vi "Create Occupancy Grid Map.vi"(8 "error in (no error)":errorcluster, 11 "occupancy grid":dbl[][](array[numeric])) -> (0 "error out":errorcluster, 3 "map reference out":refnum<data-value>)   [LabVIEW 2017, in "NI_Robotics_OccupancyGridWorldMap.lvclass"]
doc: "Generates a map in the form of a grid of variables, or cells, that describe the robot environment."
uses:
  <vilib>/robotics/Navigation/shared/WorldMap/OccupancyGridWorldMap/NI_Robotics_OccupancyGridWorldMap.lvclass
  <vilib>/robotics/Navigation/shared/MapNode/OccupancyGridNode/NI_Robotics_OccupancyGridMapNode.lvclass
  <vilib>/robotics/Navigation/shared/WorldMap/OccupancyGridWorldMap/NI_Robotics_OccupancyGridWorldMap.lvclass/NI_Robotics_OccupancyGridWorldMap.ctl
  <vilib>/robotics/Utilities/NI_Robotics Utilities.lvlib
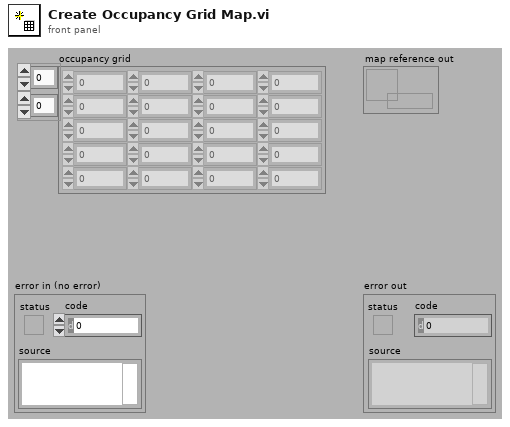
[diagram p1: front panel]
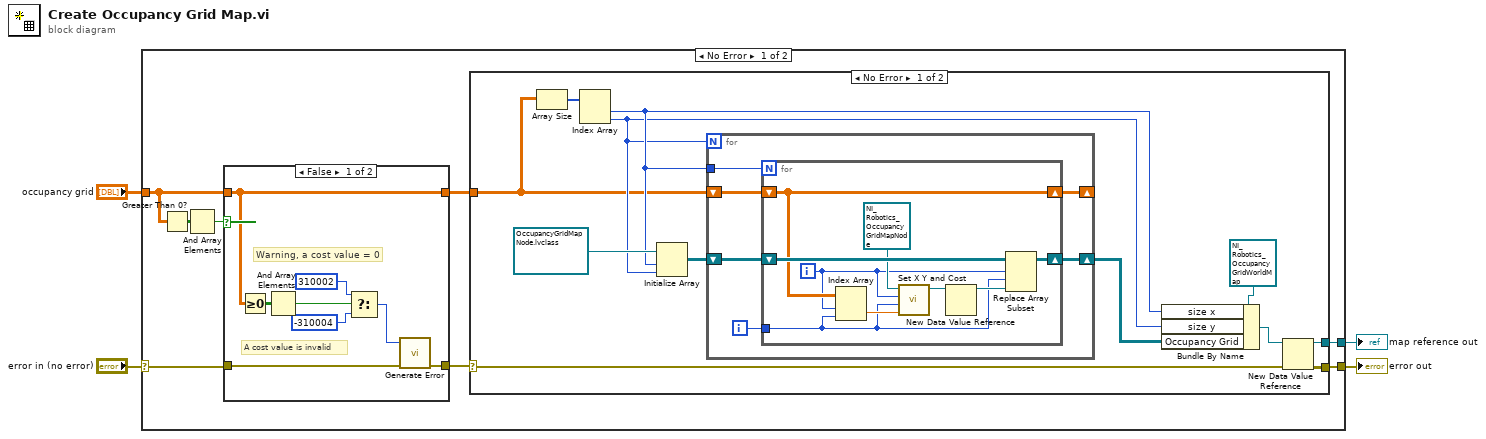
[diagram p0: block diagram]
diagram:
  n1 = case shown="No Error" "error in (no error)" {
    selector: "error in (no error)" -> [w8 w51]
    tunnel: [w11 w51] -> w1
    tunnel: "occupancy grid" -> [w5 _]
    tunnel: [w12 _] -> w2
    frame No Error {
      n2 = Greater Than 0?(x=w5) -> (x > 0?=w10:bool[][])
      n3 = And Array Elements(Boolean array=w10) -> (logical AND=w9:bool)
      n4 = case shown="False" w9 {
        tunnel: [w17 w22] -> w7
        tunnel: w8 -> [w18 w22]
        tunnel: [w13 w21] -> w6
        tunnel: w5 -> [w13 w21]
        frame False {
          # "Warning, a cost value = 0"
          # "A cost value is invalid"
          n5 = Greater Or Equal To 0?(x=w13) -> (x >= 0?=w15:bool[][])
          n6 = And Array Elements(Boolean array=w15) -> (logical AND=w14:bool)
          n7 = Select(t=310002 ("code"), s=w14, f=-310004 ("code")) -> (s? t:f=w16:i32)
          n8 = call <vilib>:"Generate Error.vi"("error in (no error)"=w18, "code"=w16) -> ("error out"=w17:errorcluster)  [unwired: 9 in]
        }
        frame True {
        }
      }
      n9 = case shown="No Error" w7 {
        selector: w7 -> [w23 w50]
        tunnel: [w29 _] -> w12
        tunnel: [w28 w50] -> w11
        tunnel: w6 -> [w24 _]
        frame No Error {
          n10 = Array Size(array=w24) -> (size(s)=w34:i32[])
          n11 = Index Array(array=w34) -> (element #1=w27:i32, element #2=w26:i32)  [unwired: 2 in]
          n12 = Initialize Array(refnum<data-value> refnum ("data value reference"), w27, w26) -> (w32:refnum<data-value>[][])
          n13 = for {
            N: w26 -> [_]
            shift-right: [w38] -> _
            shift-left: w24 -> [w39]
            tunnel: w27 -> [w40]
            shift-right: [w35] -> w31
            shift-left: w32 -> [w37]
            i -> [w36]
            n14 = for {
              N: w40 -> [_]
              shift-right: [w44] -> w38
              shift-left: w39 -> [w44]
              tunnel: w36 -> [w41]
              shift-right: [w45] -> w35
              shift-left: w37 -> [w47]
              i -> [w42]
              n15 = Index Array(array=w44, index (row)=w42, index (col)=w41) -> (element=w49:dbl)
              n16 = call-dynamic "Set X Y and Cost.vi"("Cost"=w49, "y"=w41, "x"=w42, "OccupancyGridMapNode in"=refnum<class "NI_Robotics_OccupancyGridMapNode.lvclass"> refnum) -> ("OccupancyGridMapNode out"=w48:refnum<class "NI_Robotics_OccupancyGridMapNode.lvclass">)  [unwired: 7 in]
              n17 = New Data Value Reference(data value=w48) -> (data value reference=w46:refnum<data-value>)  [unwired: 1 in, 1 out]
              n18 = Replace Array Subset(array=w47, new element=w46, index (row)=w42, index (col)=w41) -> (w45:refnum<data-value>[][])
            }
          }
          n19 = Bundle By Name(cluster=refnum<class "NI_Robotics_OccupancyGridWorldMap.lvclass"> refnum ("occupancy grid map in"), "size x"=w27, "size y"=w26, "Occupancy Grid"=w31) -> (w30:refnum<class "NI_Robotics_OccupancyGridWorldMap.lvclass">)
          n20 = New Data Value Reference(data value=w30, error in=w23) -> (data value reference=w29:refnum<data-value>, error out=w28:errorcluster)
        }
        frame Error {
        }
      }
    }
    frame Error {
    }
  }
  "error out" <- w1
  "map reference out" <- w2
